vi "Get Galaxy Locations.vi"(0 "Universe":string[][](array[string]), 1 "Galaxy (#)":string="#") -> (2 "Galaxy Locations":cdb[](array[numeric]))   [LabVIEW 2020, in "AoC 2023.lvlib"]
uses:
  AoC 2023.lvlib
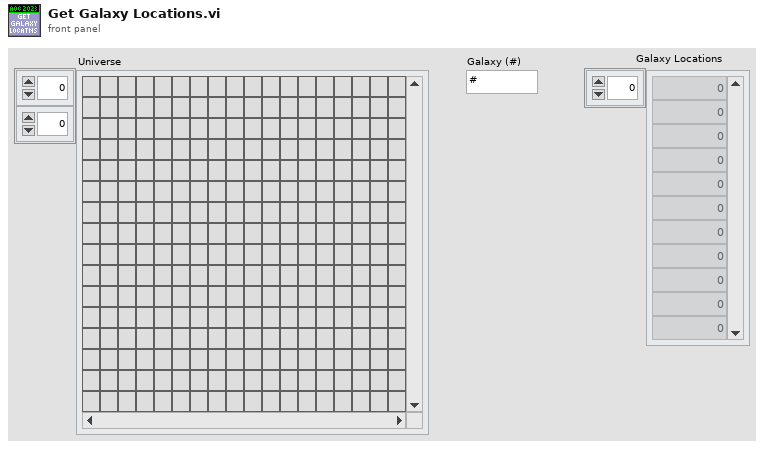
[diagram p1: front panel]
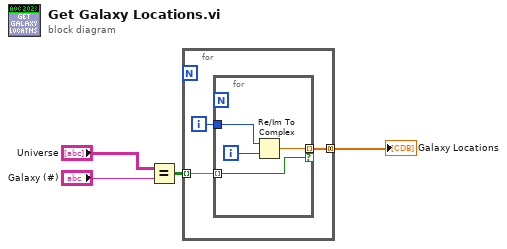
[diagram p0: block diagram]
diagram:
  n1 = Equal?(x="Universe", y="Galaxy (#)") -> (x = y?=w3:bool[][])
  n2 = for {
    tunnel: w3 -> [w7] mode=indexing
    tunnel: [w5] -> w4 mode=concatenating
    i -> [w6]
    n3 = for {
      tunnel: w7 -> [w8] mode=indexing
      tunnel: w6 -> [w11]
      tunnel: [w9] -> w5 mode=indexing if=w8
      i -> [w10]
      n4 = Re/Im To Complex(1:w10, 2:w11) -> (0:w9:cdb)
    }
  }
  "Galaxy Locations" <- w4
